vi "calibrate.vi"(8 "angle":dbl, 9 "CAD center":dbl[](array[numeric])=[100.0, 100.0], 10 "Array 3":T1(array[cluster])) -> (2 "Array 2":T1(array[cluster]))   [LabVIEW 2016]
panel:
  out "draw point Cluster in":T2
  out "draw point Cluster out":T2
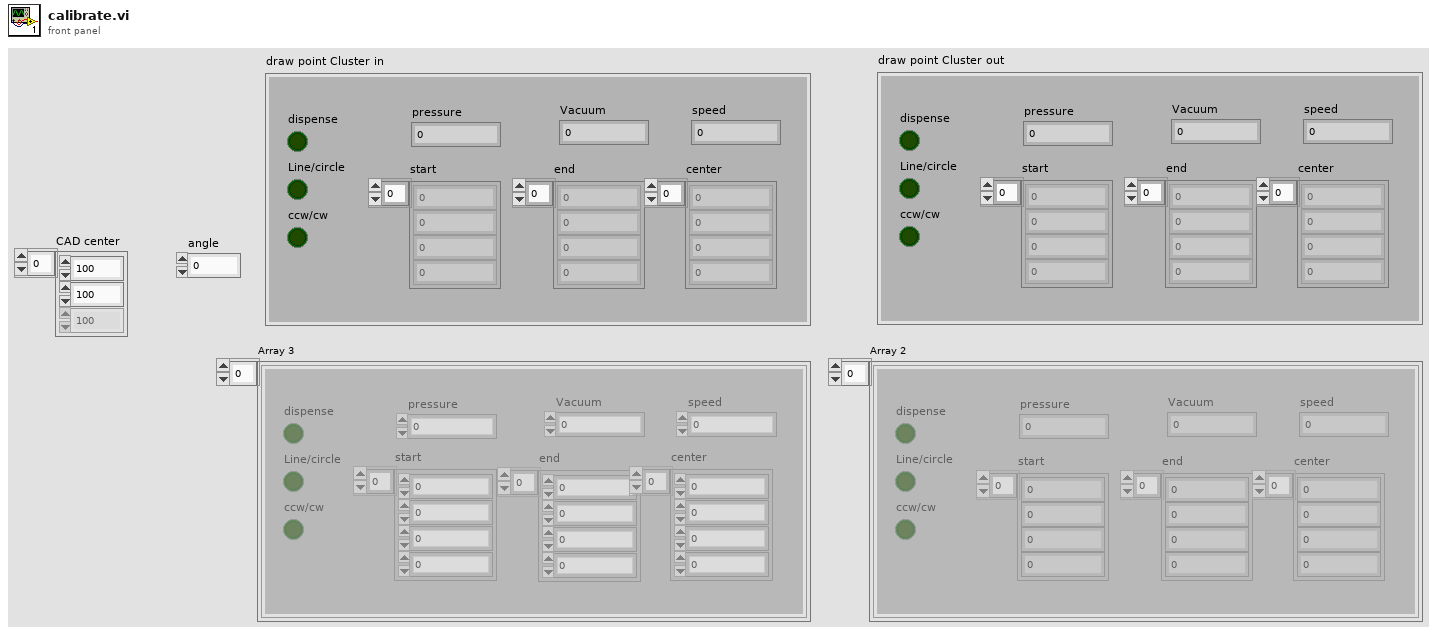
[diagram p1: front panel]
types:
  T1 = cluster{"dispense":bool, "Line/circle":bool, "ccw/cw":bool, "pressure":dbl, "speed":dbl, "start":dbl[], "end":dbl[], "center":dbl[], "Vacuum":dbl}[]
  T2 = cluster{"dispense":bool, "Line/circle":bool, "ccw/cw":bool, "pressure":dbl, "speed":dbl, "start":dbl[], "end":dbl[], "center":dbl[], "Vacuum":dbl}
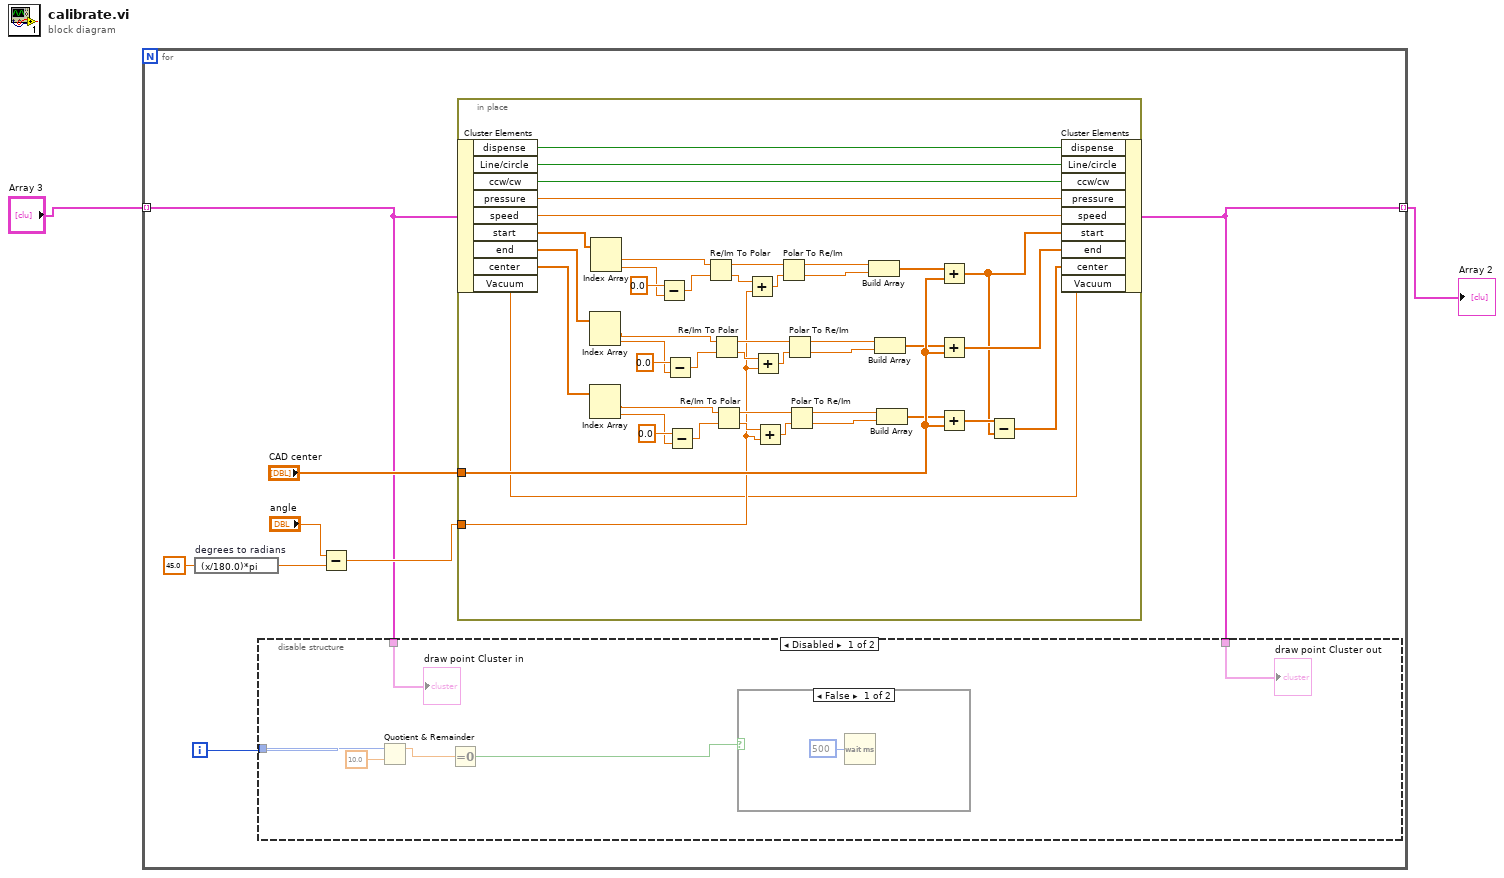
[diagram p0: block diagram]
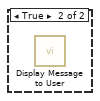
[diagram p2: hidden frame]
diagram:
  n1 = for {
    tunnel: [w10] -> w2 mode=indexing
    tunnel: "Array 3" -> [w3] mode=indexing
    i -> [w9]
    n2 = expression code="(x/180.0)*pi" "degrees to radians"(45.0) -> (w7:dbl)
    n3 = Subtract(x="angle", y=w7) -> (x-y=w5:dbl)
    n4 = in-place {
      in-place-border: "CAD center" -> [w37]
      in-place-border: w5 -> [w12]
      n5 = in-place-cluster #1(w3) -> ("dispense"=w55:bool, "Line/circle"=w54:bool, "ccw/cw"=w53:bool, "pressure"=w52:dbl, "speed"=w51:dbl, "start"=w50:dbl[], "end"=w46:dbl[], "center"=w45:dbl[], "Vacuum"=w11:dbl)
      n6 = Index Array(array=w46) -> (element #1=w17:dbl, element #2=w18:dbl)  [unwired: 2 in]
      n7 = Index Array(array=w45) -> (element #1=w16:dbl, element #2=w15:dbl)  [unwired: 2 in]
      n8 = Index Array(array=w50) -> (element #1=w34:dbl, element #2=w48:dbl)  [unwired: 2 in]
      n9 = Subtract(x=0.0, y=w48) -> (x-y=w33:dbl)
      n10 = Subtract(x=0.0, y=w18) -> (x-y=w32:dbl)
      n11 = Subtract(x=0.0, y=w15) -> (x-y=w19:dbl)
      n12 = Re/Im To Polar(2:w33, 3:w34) -> (0:w35:dbl, 1:w40:dbl)
      n13 = Re/Im To Polar(2:w32, 3:w17) -> (0:w31:dbl, 1:w27:dbl)
      n14 = Re/Im To Polar(2:w19, 3:w16) -> (0:w20:dbl, 1:w24:dbl)
      n15 = Add(x=w35, y=w12) -> (x+y=w36:dbl)
      n16 = Add(x=w31, y=w12) -> (x+y=w30:dbl)
      n17 = Add(x=w20, y=w12) -> (x+y=w21:dbl)
      n18 = Polar To Re/Im(2:w36, 3:w40) -> (0:w38:dbl, 1:w39:dbl)
      n19 = Polar To Re/Im(2:w30, 3:w27) -> (0:w29:dbl, 1:w28:dbl)
      n20 = Polar To Re/Im(2:w21, 3:w24) -> (0:w22:dbl, 1:w23:dbl)
      n21 = Build Array(w39, w38) -> (w47:dbl[])
      n22 = Build Array(w28, w29) -> (w13:dbl[])
      n23 = Build Array(w23, w22) -> (w14:dbl[])
      n24 = Add(x=w47, y=w37) -> (x+y=w42:dbl[])
      n25 = Add(x=w13, y=w37) -> (x+y=w44:dbl[])
      n26 = Add(x=w14, y=w37) -> (x+y=w43:dbl[])
      n27 = Subtract(x=w43, y=w42) -> (x-y=w41:dbl[])
      n28 = in-place-cluster #1("dispense"=w55, "Line/circle"=w54, "ccw/cw"=w53, "pressure"=w52, "speed"=w51, "start"=w42, "end"=w44, "center"=w41, "Vacuum"=w11) -> (w10:T2)
    }
    n29 = disable-structure shown="Disabled" {
      disable-tunnel: w10 -> [w56 _]
      disable-tunnel: w9 -> [w59 _]
      disable-tunnel: w3 -> [w57 _]
      frame Disabled {
        n30 = Quotient & Remainder(x=w59, y=10.0) -> (x-y*floor(x/y)=w61:dbl)  [unwired: 1 out]
        n31 = Equal To 0?(x=w61) -> (x = 0?=w58:bool)
        n32 = case shown="False" w58 {
          frame False {
            n33 = Wait (ms)(milliseconds to wait=u32 500) -> ()  [unwired: 1 out]
          }
          frame True {
            n34 = call "Display Message to User"() -> ()  [unwired: 10 in, 2 out]
          }
        }
        "draw point Cluster out" <- w56
        "draw point Cluster in" <- w57
      }
      frame Enabled {
      }
    }
  }
  "Array 2" <- w2
